vi "Main_Events Based.vi"() -> ()   [LabVIEW 2019]
doc: "This Main VI of Security System Software Demo project is developed based on User Interface Event Handler design pattern."
uses:
  Controls/Zone Status Indicators.ctl
  Controls/Module Data.ctl
panel:
  in  "Alarm Switches":bool[](array[boolean])=[FALSE, FALSE, FALSE, FALSE, FALSE, FALSE, FALSE]
  in  "Bypass Switches":bool[](array[boolean])=[FALSE, FALSE, FALSE, FALSE, FALSE, FALSE, FALSE]
  in  "Tamper Switches":bool[](array[boolean])=[FALSE, FALSE, FALSE, FALSE, FALSE, FALSE]
  out "Zone Status Indicators":T1 caption="Green    = Normal\nRed       =  Alarm\nOrange = Tamper\nBlue      = Bypass"
  in  "Stop":bool
  # "1"
  # "2"
  # "3"
  # "4"
  # "5"
  # "6"
  # "Zone"
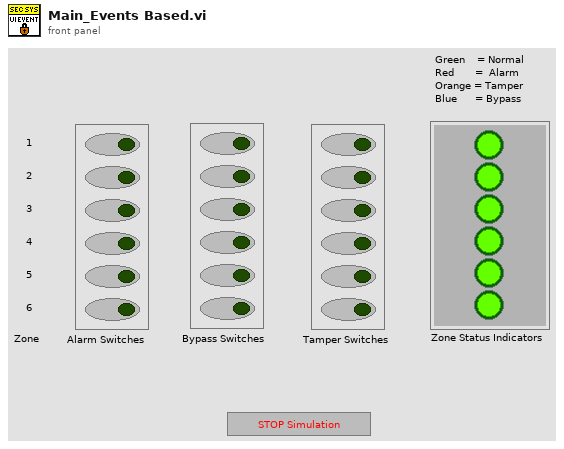
[diagram p1: front panel]
types:
  T1 = typedef "Zone Status Indicators.ctl" = cluster{"Boolean":bool, "Boolean 2":bool, "Boolean 3":bool, "Boolean 4":bool, "Boolean 5":bool, "Boolean 6":bool}
  T2 = typedef "Module Data.ctl" = cluster{"Controls[]":refnum<vi>[], "Zone Status Data":string[]}
  T3 = typedef "Zones Condition.ctl" = enum16{"Normal", "Bypass", "Tamper", "Alarm"}
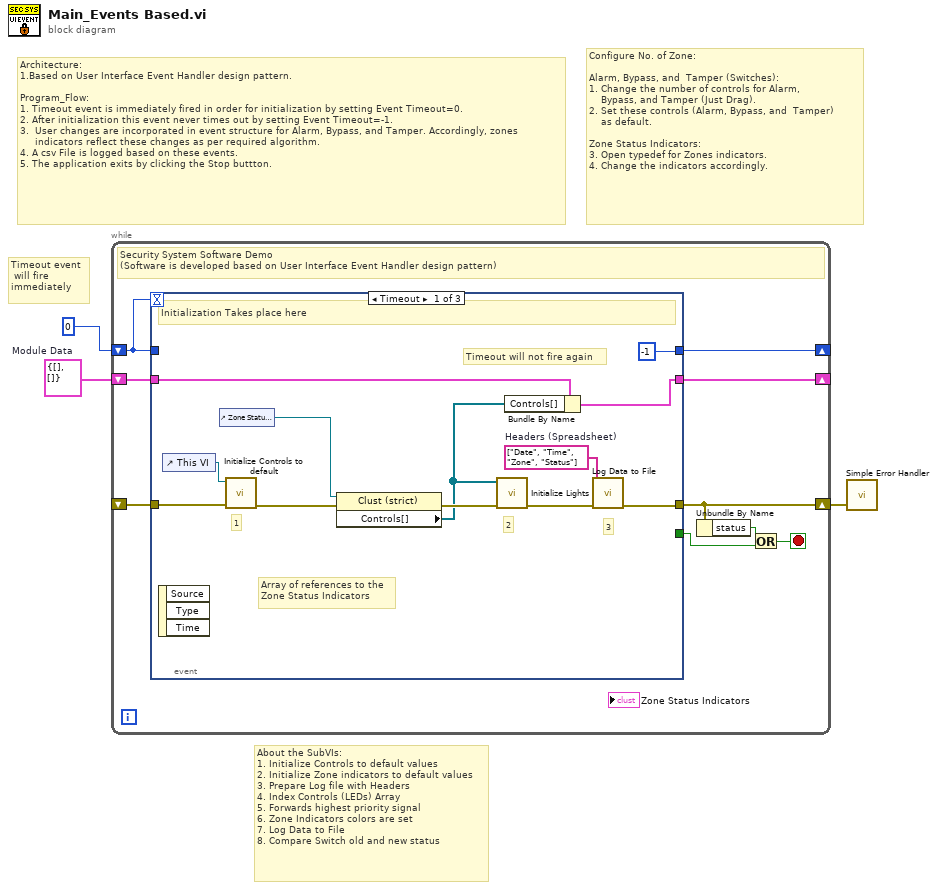
[diagram p0: block diagram]
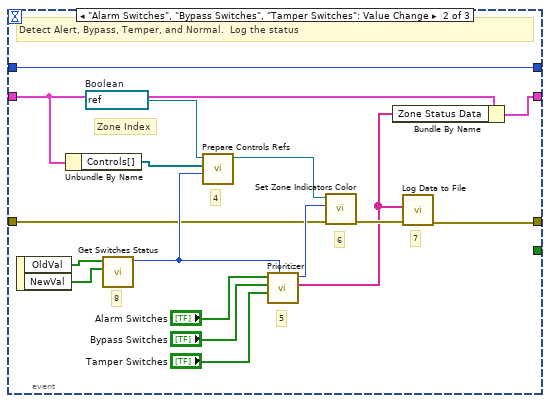
[diagram p2: hidden frame]
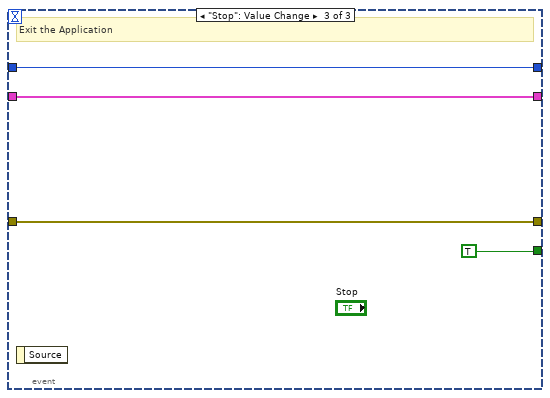
[diagram p3: hidden frame]
diagram:
  w2 = T2 {"Controls[]"=[], "Zone Status Data"=[]}  # Module Data
  # "Configure No. of Zone:\n\nAlarm, Bypass, and  Tamper (Switches):\n1. Change the number of controls for Alarm, \n    Bypass, and Tamper (Just Drag).\n2. Set these controls (Alarm, Bypass, and  Tamper) \n    as default.\n\nZone Status Indicators:\n3. Open typedef for Zones indicators.\n4. Change the indicators accordingly."
  # "About the SubVIs:\n1. Initialize Controls to default values\n2. Initialize Zone indicators to default values\n3. Prepare Log file with Headers\n4. Index Controls (LEDs) Array \n5. Forwards highest priority signal\n6. Zone Indicators colors are set\n7. Log Data to File\n8. Compare Switch old and new status"
  # "Timeout event\n will fire\nimmediately"
  # "Architecture:\n1.Based on User Interface Event Handler design pattern.  \n\nProgram_Flow:\n1. Timeout event is immediately fired in order for initialization by setting Event Timeout=0.\n2. After initialization this event never times out by setting Event Timeout=-1.\n3.  User changes are incorporated in event structure for Alarm, Bypass, and Tamper. Accordingly, zones \n     indicators reflect these changes as per required algorithm.\n4. A csv File is logged based on these events.\n5. The application exits by clicking the Stop buttton."
  n1 = while {
    shift-right: [w11] -> w3
    shift-left: _ -> [w12]
    shift-right: [w7] -> _
    shift-left: w2 -> [w6]
    shift-right: [w4] -> _
    shift-left: 0 -> [w5]
    stop <- w8 stop-if-true
    # "Security System Software Demo\n(Software is developed based on User Interface Event Handler design pattern)"
    n2 = event shown="[0] Timeout" {
      selector: _ -> [_ _ _]
      dyn-events: _ -> [_ _ _]
      timeout: w5 -> [_ _ _]
      tunnel: w12 -> [w15 w31 w45]
      tunnel: [w14 w26 w45] -> w11
      tunnel: [_ _ TRUE] -> w9
      tunnel: w6 -> [w17 w30 w44]
      tunnel: [w16 w29 w44] -> w7
      tunnel: w5 -> [_ w28 w42]
      tunnel: [-1 w28 w42] -> w4
      event Timeout {
        w22 = string[] ["Date", "Time", "Zone", "Status"]  # Headers (Spreadsheet)
        # "3"
        # "2"
        # "1"
        # "Array of references to the\nZone Status Indicators"
        # "Timeout will not fire again"
        # "Initialization Takes place here"
        n3 = event-data() -> ()  [unwired: 1 in, 3 out]
        n4 = control-ref of="This VI"() -> (w23:refnum<vi>)
        n5 = control-ref of="Zone Status Indicators"() -> (w13:refnum<vi>)
        n6 = call "Initialize Controls to default.vi"("error in (no error)"=w15, "VI in"=w23) -> ("error out"=w18:errorcluster)  [unwired: 9 in]
        n7 = property on="Property Node" class="Clust (strict)"(reference=w13, error in=w18) -> (error out=w21:errorcluster, "Controls[]"=w20:refnum<vi>[])  [unwired: 1 out]
        n8 = call "Initialize Lights.vi"("error in (no error)"=w21, "Controls[]"=w20) -> ("error out"=w19:errorcluster)  [unwired: 9 in]
        n9 = Bundle By Name(cluster=w17, "Controls[]"=w20) -> (w16:T2)
        n10 = call "Log Data to File.vi"("error in"=w19, "Log Data"=w22) -> ("error out"=w14:errorcluster)  [unwired: 9 in]
      }
      event "Alarm Switches", "Bypass Switches", "Tamper Switches": Value Change {
        w35 = refnum<vi> refnum  # Boolean
        # "8"
        # "7"
        # "6"
        # "5"
        # "4"
        # "Zone Index"
        # "Detect Alert, Bypass, Temper, and Normal.  Log the status"
        n11 = event-data() -> ("OldVal"=w41:bool[], "NewVal"=w40:bool[])  [unwired: 1 in]
        n12 = Unbundle By Name(w30) -> ("Controls[]"=w32:refnum<vi>[])
        n13 = call "Get Switches Status.vi"("NewVal"=w40, "OldVal"=w41) -> ("Zone Number - 1"=w33:i32)  [unwired: 9 in]
        n14 = call "Prepare Controls Refs.vi"("Numeric"=w33, "Controls[]"=w32, "Boolean in"=w35) -> ("Boolean out"=w34:refnum<vi>)  [unwired: 8 in]
        n15 = call "Prioritizer.vi"("Zone"=w33, "Tamper Switches"="Tamper Switches", "Bypass Switches"="Bypass Switches", "Alarm Switches"="Alarm Switches") -> ("Zone Status Data"=w25:string[], "Zone Condition"=w36:T3)  [unwired: 6 in]
        n16 = call "Set Zone Indicators Color.vi"("error in"=w31, "Alert Status"=w36, "reference"=w34) -> ("error out"=w27:errorcluster)  [unwired: 8 in]
        n17 = Bundle By Name(cluster=w30, "Zone Status Data"=w25) -> (w29:T2)
        n18 = call "Log Data to File.vi"("error in"=w27, "Log Data"=w25) -> ("error out"=w26:errorcluster)  [unwired: 9 in]
      }
      event "Stop": Value Change {
        # "Exit the Application"
        n19 = event-data() -> ()  [unwired: 1 in, 1 out]
      }
    }
    n20 = Unbundle By Name(w11) -> ("status"=w10:bool)
    n21 = Or(x=w10, y=w9) -> (x .or. y?=w8:bool)
  }
  n22 = call <vilib>:"Simple Error Handler.vi"("error in (no error)"=w3) -> ()  [unwired: 4 in, 5 out]
